vi "Get Channel TypeName from JSON Path.vi"(8 "error in":errorcluster, 11 "Path":string) -> (0 "error out":errorcluster, 3 "Type Name":string)   [LabVIEW 2026, in "NIDMM Deployment Hooks.lvlib"]
uses:
  NIDMM Deployment Hooks.lvlib
  <vilib>/regexp/Match Regular Expression.xnode
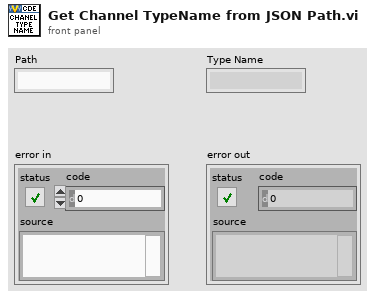
[diagram p1: front panel]
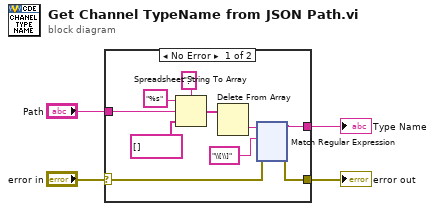
[diagram p0: block diagram]
diagram:
  n1 = case shown="No Error" "error in" {
    selector: "error in" -> [w14 w132]
    tunnel: "Path" -> [w6 _]
    tunnel: [w13 w132] -> w3
    tunnel: [w5 _] -> w1
    frame No Error {
      n2 = Spreadsheet String To Array(delimiter (Tab)=".", format string="%s", spreadsheet string=w6, array type (2D Dbl)=string[] []) -> (array=w9:string[])
      n3 = Delete From Array(array=w9) -> (deleted portion=w8:string)  [unwired: 2 in, 1 out]
      n4 = xnode "Match Regular Expression"("input string"=w8, "regular expression"="\\[\\]", "error in"=w14) -> ("before match"=w5:string, "error out"=w13:errorcluster)  [unwired: 3 in, 3 out]
    }
    frame Error {
    }
  }
  "error out" <- w3
  "Type Name" <- w1
